vi "Stuck Key Mask Parser.vi"(8 "error in (no error)":errorcluster, 10 "Parser Output Bundle":T1, 11 "Stuck Key Mask":u64) -> (0 "error out":errorcluster, 3 "output cluster":T1)   [LabVIEW 2016, in "TLMB.lvlib"]
uses:
  Projects/TLMB.lvlib
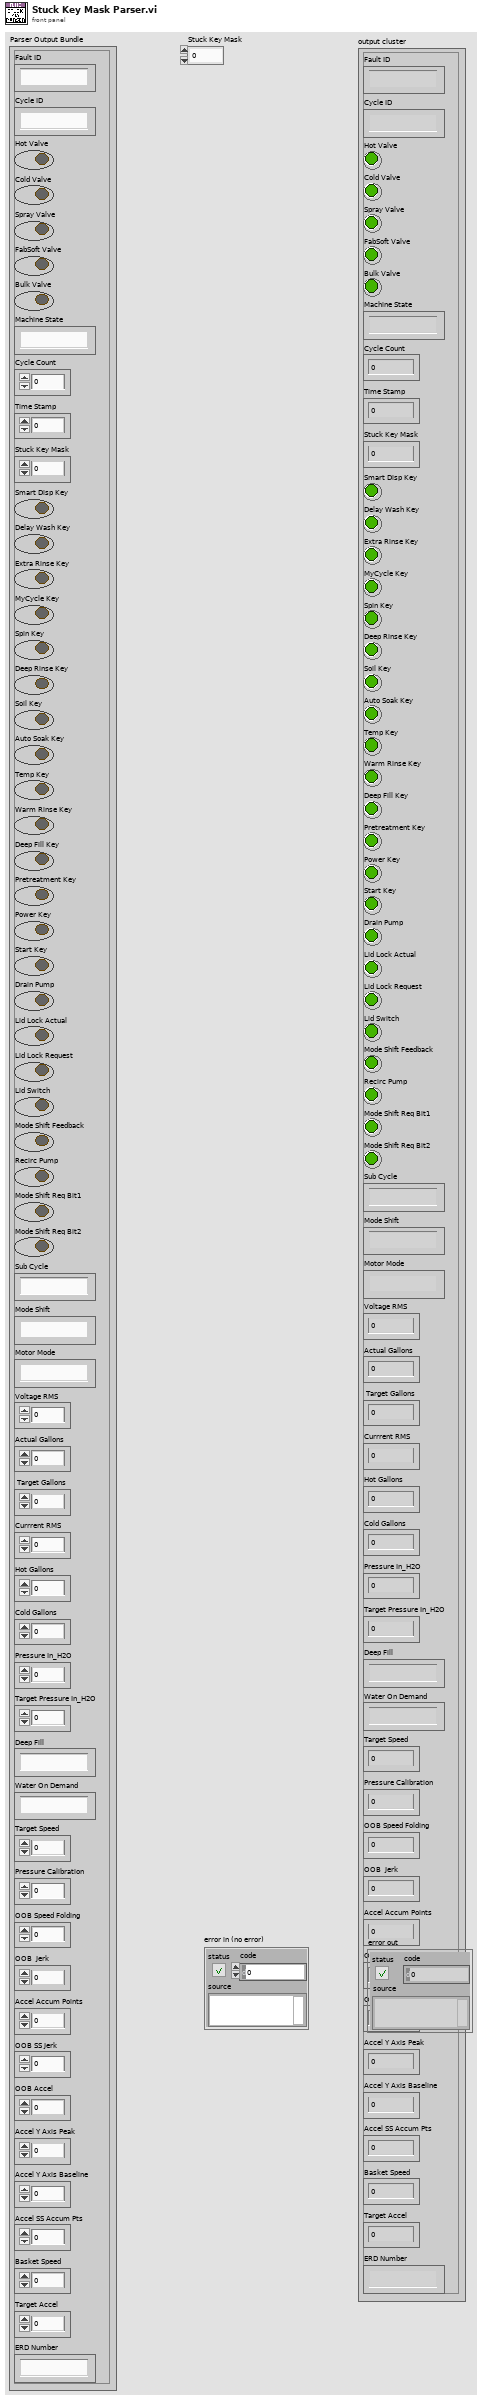
[diagram p1: front panel]
types:
  T1 = cluster{"Fault ID":string, "Cycle ID":string, "Hot Valve":bool, "Cold Valve":bool, "Spray Valve":bool, "FabSoft Valve":bool, "Bulk Valve":bool, "Machine State":string, "Cycle Count":u32, "Time Stamp":u32, "Stuck Key Mask ":u64, "Smart Disp Key":bool, "Delay Wash Key":bool, "Extra Rinse Key":bool, "MyCycle Key":bool, "Spin Key":bool, "Deep Rinse Key":bool, "Soil Key":bool, "Auto Soak Key":bool, "Temp Key":bool, "Warm Rinse Key":bool, "Deep Fill Key":bool, "Pretreatment Key":bool, "Power Key":bool, "Start Key":bool, "Drain Pump":bool, "Lid Lock Actual":bool, "Lid Lock Request":bool, "Lid Switch":bool, "Mode Shift Feedback":bool, "Recirc Pump":bool, "Mode Shift Req Bit1":bool, "Mode Shift Req Bit2":bool, "Sub Cycle":string, "Mode Shift":string, "Motor Mode":string, "Voltage RMS":u16, "Actual Gallons":u16, " Target Gallons":u16, "Currrent RMS":u16, "Hot Gallons":u16, "Cold Gallons":u16, "Pressure In_H2O":u32, "Target Pressure In_H2O":dbl, "Deep Fill":string, "Water On Demand":string, "Target Speed":u16, "Pressure Calibration":u32, "OOB Speed Folding":i32, "OOB  Jerk":i32, "Accel Accum Points":u8, "OOB SS Jerk":i32, "OOB Accel":i32, "Accel Y Axis Peak":i16, "Accel Y Axis Baseline":i16, "Accel SS Accum Pts":u8, "Basket Speed":u16, "Target Accel":u16, "ERD Number":string}
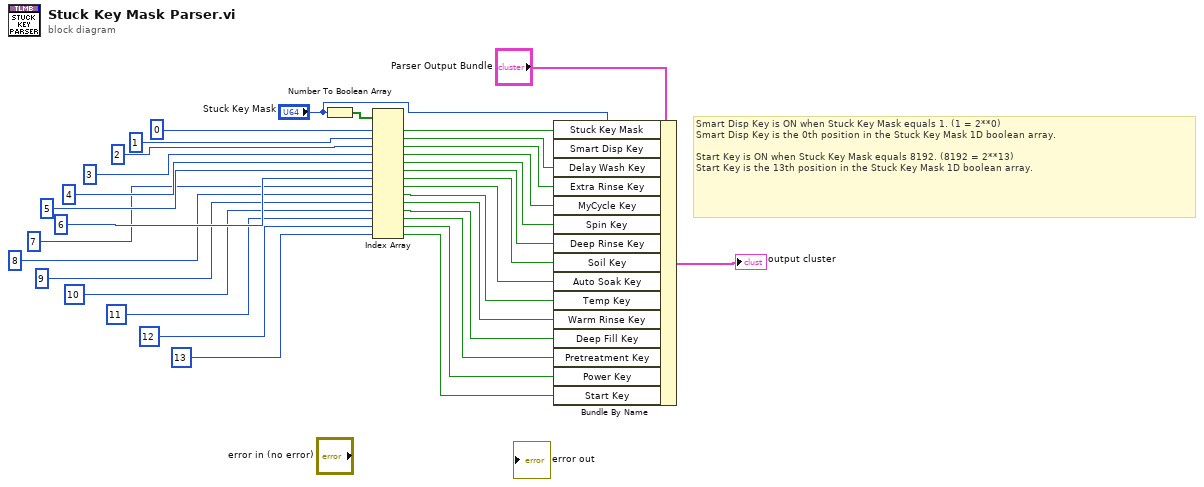
[diagram p0: block diagram]
diagram:
  # "Smart Disp Key is ON when Stuck Key Mask equals 1. (1 = 2**0)\nSmart Disp Key is the 0th position in the Stuck Key Mask 1D boolean array.\n\nStart Key is ON when Stuck Key Mask equals 8192. (8192 = 2**13)\nStart Key is the 13th position in the Stuck Key Mask 1D boolean array."
  n1 = Number To Boolean Array(number="Stuck Key Mask") -> (Boolean array=w32:bool[])
  n2 = Index Array(array=w32, index #1=0 ("index"), index #2=1 ("index"), index #3=2 ("index"), index #4=3 ("index"), index #5=4 ("index"), index #6=5 ("index"), index #7=6 ("index"), index #8=7 ("index"), index #9=8 ("index"), index #10=9 ("index"), index #11=10 ("index"), index #12=11 ("index"), index #13=12 ("index"), index #14=13 ("index")) -> (element #1=w15:bool, element #2=w14:bool, element #3=w13:bool, element #4=w12:bool, element #5=w11:bool, element #6=w10:bool, element #7=w9:bool, element #8=w8:bool, element #9=w7:bool, element #10=w6:bool, element #11=w5:bool, element #12=w4:bool, element #13=w3:bool, element #14=w2:bool)
  n3 = Bundle By Name(cluster="Parser Output Bundle", "Stuck Key Mask"="Stuck Key Mask", "Smart Disp Key"=w15, "Delay Wash Key"=w14, "Extra Rinse Key"=w13, "MyCycle Key"=w12, "Spin Key"=w11, "Deep Rinse Key"=w10, "Soil Key"=w9, "Auto Soak Key"=w8, "Temp Key"=w7, "Warm Rinse Key"=w6, "Deep Fill Key"=w5, "Pretreatment Key"=w4, "Power Key"=w3, "Start Key"=w2) -> (→"output cluster":T1)
